vi "Get Input.vi"(11 "Input ref":refnum<vi>) -> (3 "Input":string)   [LabVIEW 2023, in "AOC.lvlib"]
uses:
  AOC.lvlib
  <vilib>/Utility/error.llb/whitespace.ctl
  <vilib>/Utility/error.llb/Trim Whitespace One-Sided.vi
  <vilib>/httpClient/LabVIEWHTTPClient.lvlib
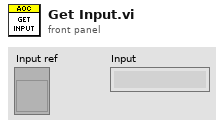
[diagram p1: front panel]
types:
  T1 = typedef "whitespace.ctl" = u16
  T2 = typedef "LabVIEWHTTPClient.lvlib/ClientHandle.ctl" = refnum<k1>
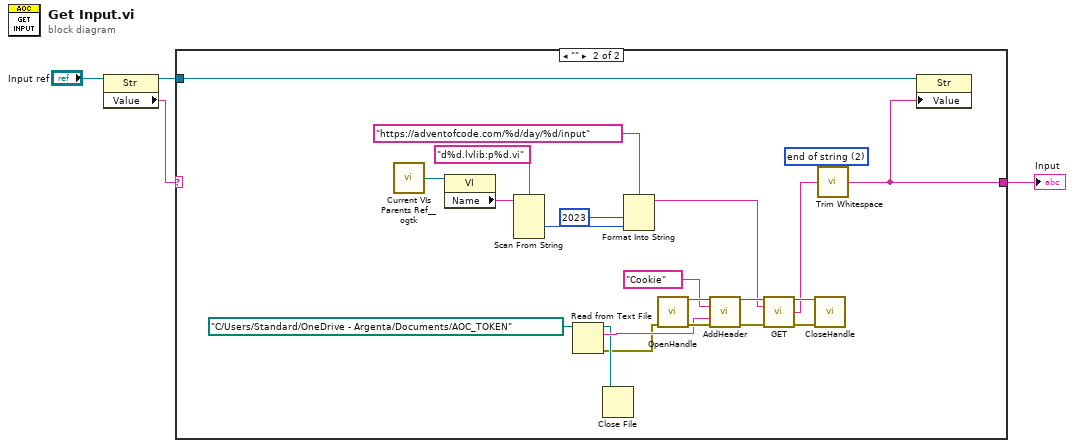
[diagram p0: block diagram]
diagram:
  n1 = property class="Str"(reference="Input ref") -> (reference out=w2:refnum<vi>, "Value"=w1:string)  [unwired: 1 in, 1 out]
  n2 = case shown="\"\"" w1 {
    selector: w1 -> [w5 _]
    tunnel: [w5 w6] -> w4
    tunnel: w2 -> [_ w9]
    frame "False", Default {
    }
    frame "" {
      w8 = T1 2 items=["both", "start of string", "end of string"] ("location (both)")
      n3 = call <userlib>:"Current VIs Parents Ref__ogtk.vi"() -> ("Calling VI's Reference"=w27:refnum<vi>)  [unwired: 2 in]
      n4 = property class="VI"(reference=w27) -> ("Name"=w11:string)  [unwired: 1 in, 2 out]
      n5 = Scan From String(format string="d%d.lvlib:p%d.vi", input string=w11) -> (output 1=w10:i32)  [unwired: 5 in, 3 out]
      n6 = Read from Text File(file (use dialog)=path "C:/Users/Standard/OneDrive - Argenta/Documents/AOC_TOKEN") -> (refnum out=w19:refnum<file>, text=w20:string, error out=w18:errorcluster)  [unwired: 3 in, 1 out]
      n7 = Close File(refnum=w19) -> ()  [unwired: 1 in, 2 out]
      n8 = Format Into String(format string="https://adventofcode.com/%d/day/%d/input", 2023, w10) -> (resulting string=w15:string)  [unwired: 2 in, 1 out]
      n9 = call <vilib>:"OpenHandle.vi"("error in (no error)"=w18) -> ("client handle out"=w25:T2, "error out"=w24:errorcluster)  [unwired: 13 in]
      n10 = call <vilib>:"AddHeader.vi"("client handle"=w25, "header"="Cookie", "value"=w20, "error in (no error)"=w24) -> ("client handle out"=w17:T2, "error out"=w16:errorcluster)  [unwired: 10 in]
      n11 = call <vilib>:"GET.vi"("client handle"=w17, "url"=w15, "error in (no error)"=w16) -> ("client handle out"=w13:T2, "body"=w7:string, "error out"=w12:errorcluster)  [unwired: 9 in, 1 out]
      n12 = call <vilib>:"CloseHandle.vi"("client handle"=w13, "error in (no error)"=w12) -> ()  [unwired: 13 in, 1 out]
      n13 = call <vilib>:"Trim Whitespace.vi"("string"=w7, "location (both)"=w8) -> ("trimmed string"=w6:string)
      n14 = property on="Property Node" class="Str"(reference=w9, "Value"=w6) -> ()  [unwired: 1 in, 2 out]
    }
  }
  "Input" <- w4
